vi "Actor Core.vi"(8 "error in":errorcluster, 11 "BNT_DSCXtGraph in":refnum<class "BNT_DSCXtGraph.lvclass">) -> (0 "error out":errorcluster, 3 "Actor out":refnum<class "Actor.lvclass">)   [LabVIEW 2021, in "BNT_DSCXtGraph.lvlib" / "BNT_DSCXtGraph.lvclass"]
doc: "(<B>Filename</B>: Actor Framework.lvlib:Actor.lvclass:Actor Core.vi)\n\nReceives messages to the actor, reacts to them, and initiates any error handling that may shut the actor down.\n\nDescendant classes may override this VI to append parallel tasks for the actor to complete while it handles messages. Overrides use the Call Parent Method node."
uses:
  BNT_DSCXtGraph.lvclass
  C:/Users/Holger/Documents/LVP/BNT/EQCR/Packages/CSPP_Core/Actors/CSPP_BaseActor/CSPP_BaseActor.lvclass
  C:/Program Files (x86)/National Instruments/LabVIEW 2021/vi.lib/ActorFramework/Actor/Actor.lvclass
  C:/Users/Holger/Documents/LVP/BNT/EQCR/Packages/CSPP_Core/Actors/CSPP_GUIActor/CSPP_GUIActor.lvclass
  <vilib>/ActorFramework/Actor/Actor.lvclass
  CSPP_Core/Actors/CSPP_BaseActor/CSPP_BaseActor.lvclass/CSPP_BaseActor.ctl
  BNT_DSCXtGraph.lvclass/BNT_DSCXtGraph.ctl
  <vilib>/ActorFramework/Actor/Actor.lvclass/Actor.ctl
  <vilib>/ActorFramework/Message Enqueuer/Message Enqueuer.lvclass/Message Enqueuer.ctl
  CSPP_Core/Actors/CSPP_GUIActor/CSPP_GUIActor.lvclass/CSPP_GUIActor.ctl
  BNT_DSCXtGraph Messages/Trace Query Options Msg/Trace Query Options Msg.lvclass/Trace Query Options Msg.ctl
  CSPP_Core/Actors/CSPP_BaseActor/Read Object Name.vi
  CSPP_Core/Actors/CSPP_GUIActor/Read Stop-Event.vi
  CSPP_Core/Actors/CSPP_GUIActor/Read PV-Update.vi
  <vilib>/ActorFramework/Message Enqueuer/Init from Existing Queue.vi
  <vilib>/ActorFramework/Message Enqueuer/Enqueue.vi
  BNT_DSCXtGraph Messages/Read Decimated Traces Msg/Read Decimated Traces Msg.lvclass
  C:/Program Files (x86)/National Instruments/LabVIEW 2021/vi.lib/ActorFramework/Message/Message.lvclass
  <vilib>/ActorFramework/Stop Msg/Stop Msg.lvclass
  BNT_DSCXtGraph Messages/Trace Query Options Msg/Trace Query Options Msg.lvclass
  <vilib>/ActorFramework/Message Priority Queue/Priority Enqueue.vi
  <vilib>/ActorFramework/Message Enqueuer/Message Enqueuer.lvclass
  CSPP_Core/Classes/CSPP_ProcessVariables/ProcessVariable/PV.lvclass
  CSPP_Core/Actors/CSPP_GUIActor/CSPP_GUIActor.lvclass
  CSPP_Core/Actors/CSPP_BaseActor/CSPP_BaseActor.lvclass
  CSPP_Core/Libraries/Utilities/CSPP_Utilities.lvlib
panel:
  out "XY Graph":T1(graph)
  in  "Stop Button":bool
  in  "Start Time":timestamp format="%<%H:%M:%S\n%Y/%m/%d>T"
  in  "Max Points per Trace (-1:all)":i32=-1
  in  "Options":T2={"interpolate data (F)"=FALSE, "extrapolate to now (F)"=FALSE, "remove data breaks (F)"=FALSE, "interpolation interval (1 s)"=1.0, "maintain trending info (T)"=TRUE} {"interpolation interval (1 s)" min=0.0 format="%0.2f"}
  in  "Stop Time":timestamp format="%<%H:%M:%S\n%Y/%m/%d>T"
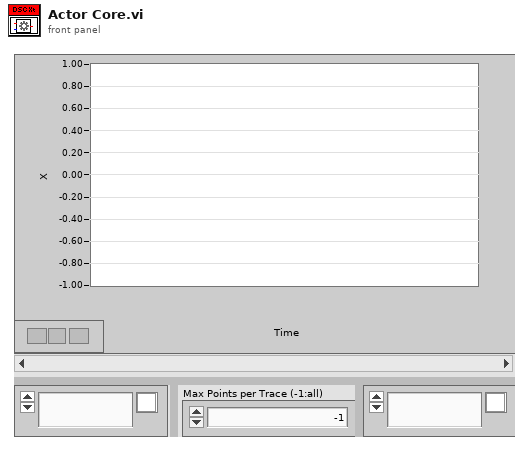
[diagram p1: front panel]
types:
  T1 = cluster{"timestamps":timestamp[], "data":dbl[]}[]
  T2 = cluster{"interpolate data (F)":bool, "extrapolate to now (F)":bool, "remove data breaks (F)":bool, "interpolation interval (1 s)":dbl, "maintain trending info (T)":bool}
  T3 = enum32{"Invalid", "Standard", "Closed", "Hidden", "Minimized", "Maximized"}
  T4 = cluster{"Start Time":timestamp, "Stop Time":timestamp}
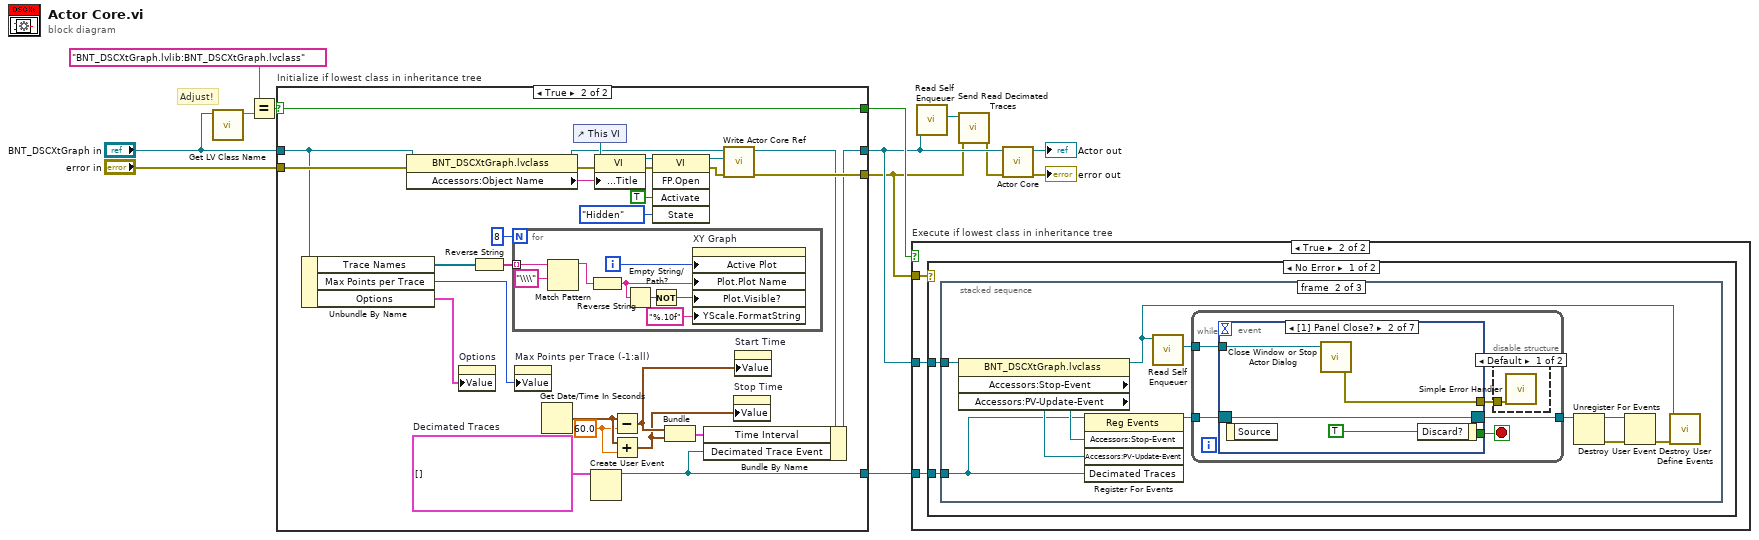
[diagram p0: block diagram]
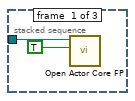
[diagram p3: hidden frame]
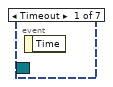
[diagram p4: hidden frame]
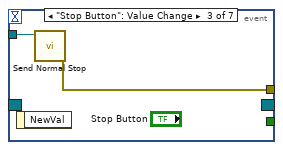
[diagram p5: hidden frame]
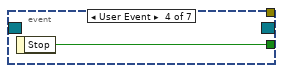
[diagram p6: hidden frame]
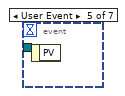
[diagram p7: hidden frame]
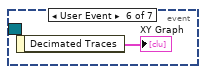
[diagram p8: hidden frame]
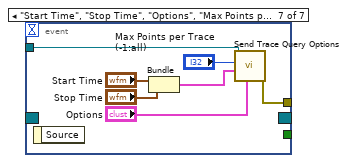
[diagram p9: hidden frame]
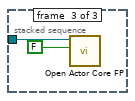
[diagram p11: hidden frame]
diagram:
  # "Adjust!"
  n1 = call <vilib>:"Get LV Class Name.vi"("object"="BNT_DSCXtGraph in") -> ("class name"=w13:string)  [unwired: 9 in, 1 out]
  n2 = Equal?(x="BNT_DSCXtGraph.lvlib:BNT_DSCXtGraph.lvclass" ("class name"), y=w13) -> (x = y?=w11:bool)
  n3 = case "Initialize if lowest class in inheritance tree" shown="True" w11 {
    selector: w11 -> [w16 w42]
    tunnel: "error in" -> [w14 w40]
    tunnel: "BNT_DSCXtGraph in" -> [w15 w31]
    tunnel: [w15 w27] -> w8
    tunnel: [w14 w38] -> w2
    tunnel: [w16 w42] -> w10
    tunnel: [_ w26] -> w9
    frame False {
    }
    frame True {
      w23 = 60.0
      w25 = T1 []  # Decimated Traces
      n4 = Unbundle By Name(w31) -> ("Trace Names"=w29:refnum<k21>[], "Max Points per Trace"=w19:i32, "Options"=w18:T2)
      n5 = property class="BNT_DSCXtGraph.lvclass"(reference=w31, error in=w40) -> (reference out=w32:refnum<class "BNT_DSCXtGraph.lvclass">, error out=w34:errorcluster, "Accessors:Object Name"=w33:string)
      n6 = property on="Options" class="Clust (strict)"("Value"=w18) -> ()  [unwired: 2 in, 2 out]
      n7 = Reverse String(1:w29) -> (0:w30:string[])
      n8 = for {
        N: 8 -> [_]
        tunnel: w30 -> [w52] mode=indexing
        i -> [w49]
        n9 = Match Pattern(string=w52, regular expression="\\\\") -> (before substring=w50:string)  [unwired: 1 in, 3 out]
        n10 = Reverse String(1:w50) -> (0:w47:string)
        n11 = Empty String/Path?(string/path=w47) -> (empty?=w46:bool)
        n12 = Not(x=w46) -> (.not. x?=w48:bool)
        n13 = property on="XY Graph" class="XYGraph (strict)"("Active Plot"=w49, "Plot.Plot Name"=w47, "Plot.Visible?"=w48, "YScale.FormatString"="%.10f" ("Y Scale.Format String")) -> ()  [unwired: 2 in, 2 out]
      }
      n14 = property on="Max Points per Trace (-1:all)" class="DigNum (strict)"("Value"=w19) -> ()  [unwired: 2 in, 2 out]
      n15 = Get Date/Time In Seconds() -> (seconds since 1Jan1904=w24:timestamp)
      n16 = control-ref of="This VI"() -> (w37:refnum<vi>)
      n17 = Create User Event(user event datatype=w25) -> (user event=w26:refnum<user-event>)  [unwired: 1 in, 1 out]
      n18 = property class="VI"(reference=w37, error in=w34, "Front Panel.Title"=w33) -> (reference out=w36:refnum<vi>, error out=w35:errorcluster)
      n19 = Subtract(x=w24, y=w23) -> (x-y=w21:timestamp)
      n20 = Add(x=w24, y=w23) -> (x+y=w20:timestamp)
      n21 = invoke class="VI" method="FP.Open"(reference=w36, error in=w35, "Activate"=TRUE ("Activate?"), "State"=T3."Hidden") -> (reference out=w41:refnum<vi>, error out=w39:errorcluster)  [unwired: 1 in, 3 out]
      n22 = Bundle(w21, w20) -> (w22:cluster{timestamp, timestamp})  [unwired: 1 in]
      n23 = call "Write Actor Core Ref.vi"("error in (no error)"=w39, "Actor Core Ref"=w41, "CSPP_BaseActor in"=w32) -> ("error out"=w38:errorcluster, "CSPP_BaseActor out"=w28:refnum<class "BNT_DSCXtGraph.lvclass">)  [unwired: 7 in]
      n24 = Bundle By Name(cluster=w28, "Time Interval"=w22, "Decimated Trace Event"=w26) -> (w27:refnum<class "BNT_DSCXtGraph.lvclass">)
      n25 = property on="Stop Time" class="AbsTime (strict)"("Value"=w20) -> ()  [unwired: 2 in, 2 out]
      n26 = property on="Start Time" class="AbsTime (strict)"("Value"=w21) -> ()  [unwired: 2 in, 2 out]
    }
  }
  n27 = case "Execute if lowest class in inheritance tree" shown="True" w10 {
    tunnel: w8 -> [_ w55]
    tunnel: w2 -> [_ w54]
    tunnel: w9 -> [_ w53]
    frame False {
    }
    frame True {
      n28 = case shown="No Error" w54 {
        tunnel: w55 -> [w57 _]
        tunnel: w53 -> [w56 _]
        frame No Error {
          n29 = stacked-sequence {
            tunnel: w57 -> [w59 w69 w91]
            tunnel: w56 -> [_ w60 _]
            frame #0 {
              n30 = call "Open Actor Core FP.vi"("Open FP (F)"=TRUE, "CSPP_BaseActor in"=w59) -> ()  [unwired: 8 in, 2 out]
            }
            frame #1 {
              n31 = property class="BNT_DSCXtGraph.lvclass"(reference=w69) -> (reference out=w67:refnum<class "BNT_DSCXtGraph.lvclass">, "Accessors:Stop-Event"=w64:refnum<user-event>, "Accessors:PV-Update-Event"=w63:refnum<user-event>)  [unwired: 1 in, 1 out]
              n32 = register-events(w64, w63, w60) -> (reference out=w65:refnum<event-registration>)  [unwired: 2 in, 1 out]
              n33 = call <vilib>:"Read Self Enqueuer.vi"("Actor"=w67) -> ("Self Enqueuer"=w66:refnum<class "Message Enqueuer.lvclass">)  [unwired: 10 in]
              n34 = while {
                tunnel: w65 -> [w74]
                tunnel: [w72] -> w68
                tunnel: w66 -> [w70]
                stop <- w73 stop-if-true
                n35 = event shown="[1] Panel Close?" {
                  selector: w74 -> [_ _ _ _ _ _ _]
                  dyn-events: [_ _ _ _ _ _ _] -> w72
                  timeout: _ -> [_ _ _ _ _ _ _]
                  tunnel: [_ _ _ w80 _ _ _] -> w73
                  tunnel: [_ w75 w79 _ _ _ w86] -> w71
                  tunnel: w70 -> [_ w76 w78 _ _ _ w88]
                  event Timeout {
                    n36 = event-data() -> ()  [unwired: 1 in, 1 out]
                  }
                  event Panel Close? {
                    n37 = event-data() -> ()  [unwired: 1 in, 1 out]
                    n38 = call "Close Window or Stop Actor Dialog.vi"("Self Enqueuer"=w76) -> ("Error Out"=w75:errorcluster)  [unwired: 2 in]
                    n39 = event-data("Discard?"=TRUE) -> ()  [unwired: 1 in, 1 out]
                  }
                  event "Stop Button": Value Change {
                    n40 = event-data() -> ()  [unwired: 1 in, 1 out]
                    n41 = call <vilib>:"Send Normal Stop.vi"("Message Enqueuer"=w78) -> ("error out"=w79:errorcluster)  [unwired: 10 in]
                  }
                  event User Event {
                    n42 = event-data() -> ("Stop"=w80:bool)  [unwired: 1 in]
                  }
                  event User Event {
                    n43 = event-data() -> ()  [unwired: 1 in, 1 out]
                  }
                  event User Event {
                    n44 = event-data() -> ("Decimated Traces"=→"XY Graph":T1)  [unwired: 1 in]
                  }
                  event "Start Time", "Stop Time", "Options", "Max Points per Trace (-1:all)": Value Change {
                    n45 = event-data() -> ()  [unwired: 1 in, 1 out]
                    n46 = Bundle("Start Time"="Start Time", "Stop Time"="Stop Time") -> (w82:T4)  [unwired: 1 in]
                    n47 = call "Send Trace Query Options.vi"("Options"="Options", "Time Interval"=w82, "Max Points per Trace (all)"="Max Points per Trace (-1:all)", "Message Enqueuer"=w88) -> ("error out"=w86:errorcluster)  [unwired: 6 in, 1 out]
                  }
                }
                n48 = disable-structure shown="Default" {
                  disable-tunnel: w71 -> [w89 _]
                  frame condition #0 (active) {
                    n49 = call <vilib>:"Simple Error Handler.vi"("error in (no error)"=w89) -> ()  [unwired: 4 in, 5 out]
                  }
                  frame condition #1 {
                  }
                }
              }
              n50 = Unregister For Events(event registration refnum=w68) -> (error out=w62:errorcluster)  [unwired: 1 in]
              n51 = Destroy User Event(user event=w60, error in=w62) -> (error out=w61:errorcluster)
              n52 = call-dynamic "Destroy User Define Events.vi"("error in (no error)"=w61, "CSPP_GUIActor in"=w67) -> ()  [unwired: 8 in, 2 out]
            }
            frame #2 {
              n53 = call "Open Actor Core FP.vi"("Open FP (F)"=FALSE, "CSPP_BaseActor in"=w91) -> ()  [unwired: 8 in, 2 out]
            }
          }
        }
        frame Error {
        }
      }
    }
  }
  n54 = call <vilib>:"Read Self Enqueuer.vi"("Actor"=w8) -> ("Self Enqueuer"=w3:refnum<class "Message Enqueuer.lvclass">)  [unwired: 10 in]
  n55 = call "Send Read Decimated Traces.vi"("error in (no error)"=w2, "Message Enqueuer"=w3) -> ("error out"=w1:errorcluster)  [unwired: 8 in, 1 out]
  n56 = call-parent "Actor Core.vi"("error in"=w1, "CSPP_GUIActor in"=w8) -> ("error out"=→"error out":errorcluster, "Actor out"=→"Actor out":refnum<class "Actor.lvclass">)  [unwired: 8 in]
